vi "configDAQmx.vi"(8 "error in (no error)":errorcluster, 10 "DAQ.Config":T1={"Channels"="", "DAQ_Type"=enum."AI", "minimum value"=-5.0, "maximum value"=5.0, "DAQ_SamplingInfo"={"Fs"=1000.0, "#s"=1000.0}, "DAQ_SamplingMode"=enum."Continuous"} {"maximum value" format="%0.2f"; "minimum value" format="%0.2f"}, 11 "DAQmx in":refnum<class "DAQmx.lvclass">) -> (0 "error out":errorcluster, 3 "DAQmx out":refnum<class "DAQmx.lvclass">)   [LabVIEW 2016, in "DAQmx.lvclass"]
uses:
  DAQmx.lvclass
  C:/user/patrick/hg/lockin.SMO/lvsrc/SMOs/DAQ/DAQ.lvclass
  DAQ/Typedefs/DAQ_Config.ctl
  DAQ/Typedefs/PrivateEvents--DAQ.AI.Channels.ctl
  DAQ/Typedefs/DAQ_Type.ctl
  DAQ/Typedefs/DAQ_SamplingInfo.ctl
  DAQ/Typedefs/DAQ_SamplingMode.ctl
  DAQmx.lvclass/DAQmx.ctl
  DAQ/DAQ.lvclass
panel:
  # "Specific DAQmx config\nWire it to the connector pane"
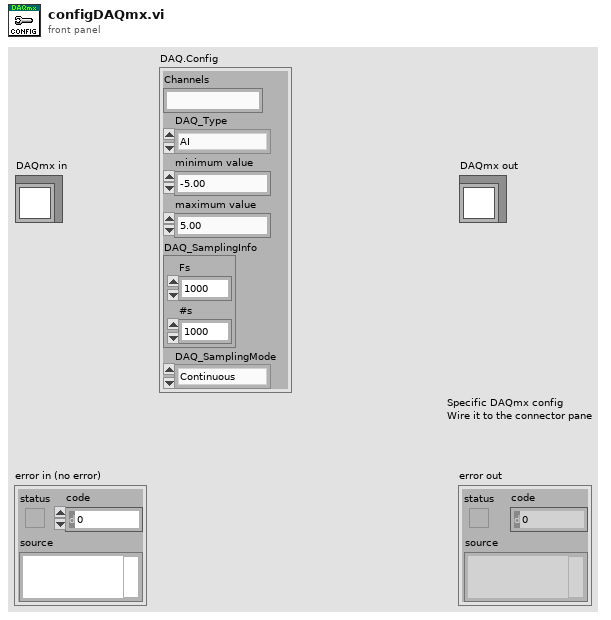
[diagram p1: front panel]
types:
  T1 = typedef "DAQ.lvclass/DAQ_Config.ctl" = cluster{"Channels":T2, "DAQ_Type":T3, "minimum value":dbl, "maximum value":dbl, "DAQ_SamplingInfo":T4, "DAQ_SamplingMode":T5}
  T2 = typedef "DAQ.lvclass/PrivateEvents--DAQ.AI.Channels.ctl" = string
  T3 = typedef "DAQ.lvclass/DAQ_Type.ctl" = enum16{"AI", "AO"}
  T4 = typedef "DAQ.lvclass/DAQ_SamplingInfo.ctl" = cluster{"Fs":dbl, "#s":dbl}
  T5 = typedef "DAQ.lvclass/DAQ_SamplingMode.ctl" = enum16{"Continuous", "Finite"}
  T6 = typedef "DAQmx.lvclass/DAQmx_Config.ctl" = cluster{"Buffer Size (S)":i32, "Master Slave":enum16{"MASTER", "SLAVE"}}
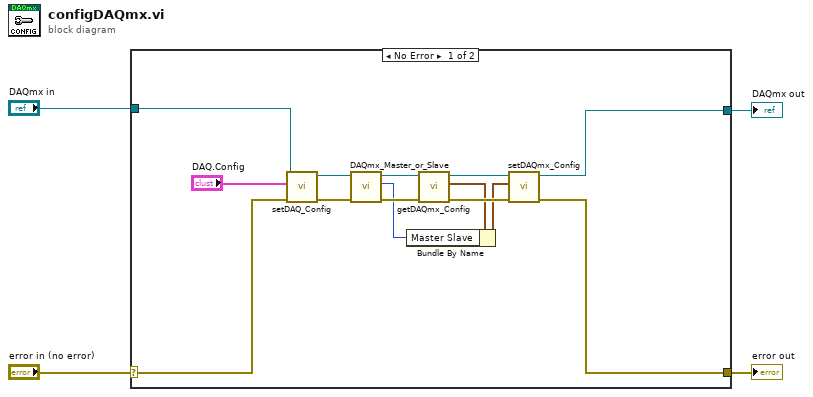
[diagram p0: block diagram]
diagram:
  n1 = case shown="No Error" "error in (no error)" {
    selector: "error in (no error)" -> [w14 w20]
    tunnel: [w5 w20] -> w3
    tunnel: [w6 w19] -> w1
    tunnel: "DAQmx in" -> [w18 w19]
    frame No Error {
      n2 = call "setDAQ_Config.vi"("error in (no error)"=w14, "DAQ.Config"="DAQ.Config", "DAQ in"=w18) -> ("error out"=w15:errorcluster, "DAQ out"=w16:refnum<class "DAQmx.lvclass">)  [unwired: 7 in]
      n3 = call "DAQmx_Master_or_Slave.vi"("error in (no error)"=w15, "DAQmx in"=w16) -> ("error out"=w13:errorcluster, "Enum"=w7:enum16{"MASTER", "SLAVE"}, "DAQmx out"=w12:refnum<class "DAQmx.lvclass">)  [unwired: 7 in]
      n4 = call "getDAQmx_Config.vi"("error in (no error)"=w13, "DAQmx in"=w12) -> ("error out"=w10:errorcluster, "DAQmx.Config"=w9:T6, "DAQmx out"=w11:refnum<class "DAQmx.lvclass">)  [unwired: 7 in]
      n5 = Bundle By Name(cluster=w9, "Master Slave"=w7) -> (w8:T6)
      n6 = call "setDAQmx_Config.vi"("error in (no error)"=w10, "DAQmx.Config"=w8, "DAQmx in"=w11) -> ("error out"=w5:errorcluster, "DAQmx out"=w6:refnum<class "DAQmx.lvclass">)  [unwired: 7 in]
    }
    frame Error {
    }
  }
  "error out" <- w3
  "DAQmx out" <- w1
